vi "GenTargetGait.vi"() -> ()   [LabVIEW 2016]
uses:
  Sim&Process/DataProcess/CAlex2-Data/CAlex2_Data.lvclass
  D:/JinXin/LabVIEW.git/CAlex2-Controller-master/Sim&Process/DataProcess/ExpData/ExpData.lvclass
  Sim&Process/DataProcess/CAlex2-Data/PropertyNodes/Get_JointAngles.vi
  <vilib>/Utility/file.llb/Write Delimited Spreadsheet (string).vi
  <vilib>/Utility/file.llb/Write Delimited Spreadsheet (DBL).vi
  Sim&Process/DataProcess/ExpData/ExpData.lvclass
  <vilib>/GoldZinc Software/auzn custom VIs/CustomVI.lvlib
panel:
  out "AveragedJointAngle":dbl[][](array[numeric])
  out "TargetJointAngle":dbl[][](array[numeric])
  out "TargetTraj":dbl[][](array[numeric])
  in  "Save":bool
  in  "ScalingCoef Knee":dbl=1.0 format="%#_13g"
  out "Leg Length":cluster{"Thigh":dbl, "Shank":dbl}
  in  "Scale Method":enum16{"GaitHeight", "Angle"}(ring)
  in  "OutputLength":i32=500
  in  "ScalingCoef Hip":dbl=1.3 format="%#_13g"
  out "Array":dbl[](array[numeric])
  in  "Update":bool
  in  "Open":bool
  in  "stop":bool
  in  "EndTime":dbl=240.0
  in  "StartTime":dbl=60.0
  in  "Cut":bool
  out "AveragedTrajectory":dbl[][](graph)
  out "Averaged":cluster{"Mean":dbl[], "Mean":dbl[]}[](graph)
  out "Stacked":T1(graph)
  out "Ankle - X":dbl[][](graph)
  in  "Cut Parameter":dbl=100.0
  in  "Path":path
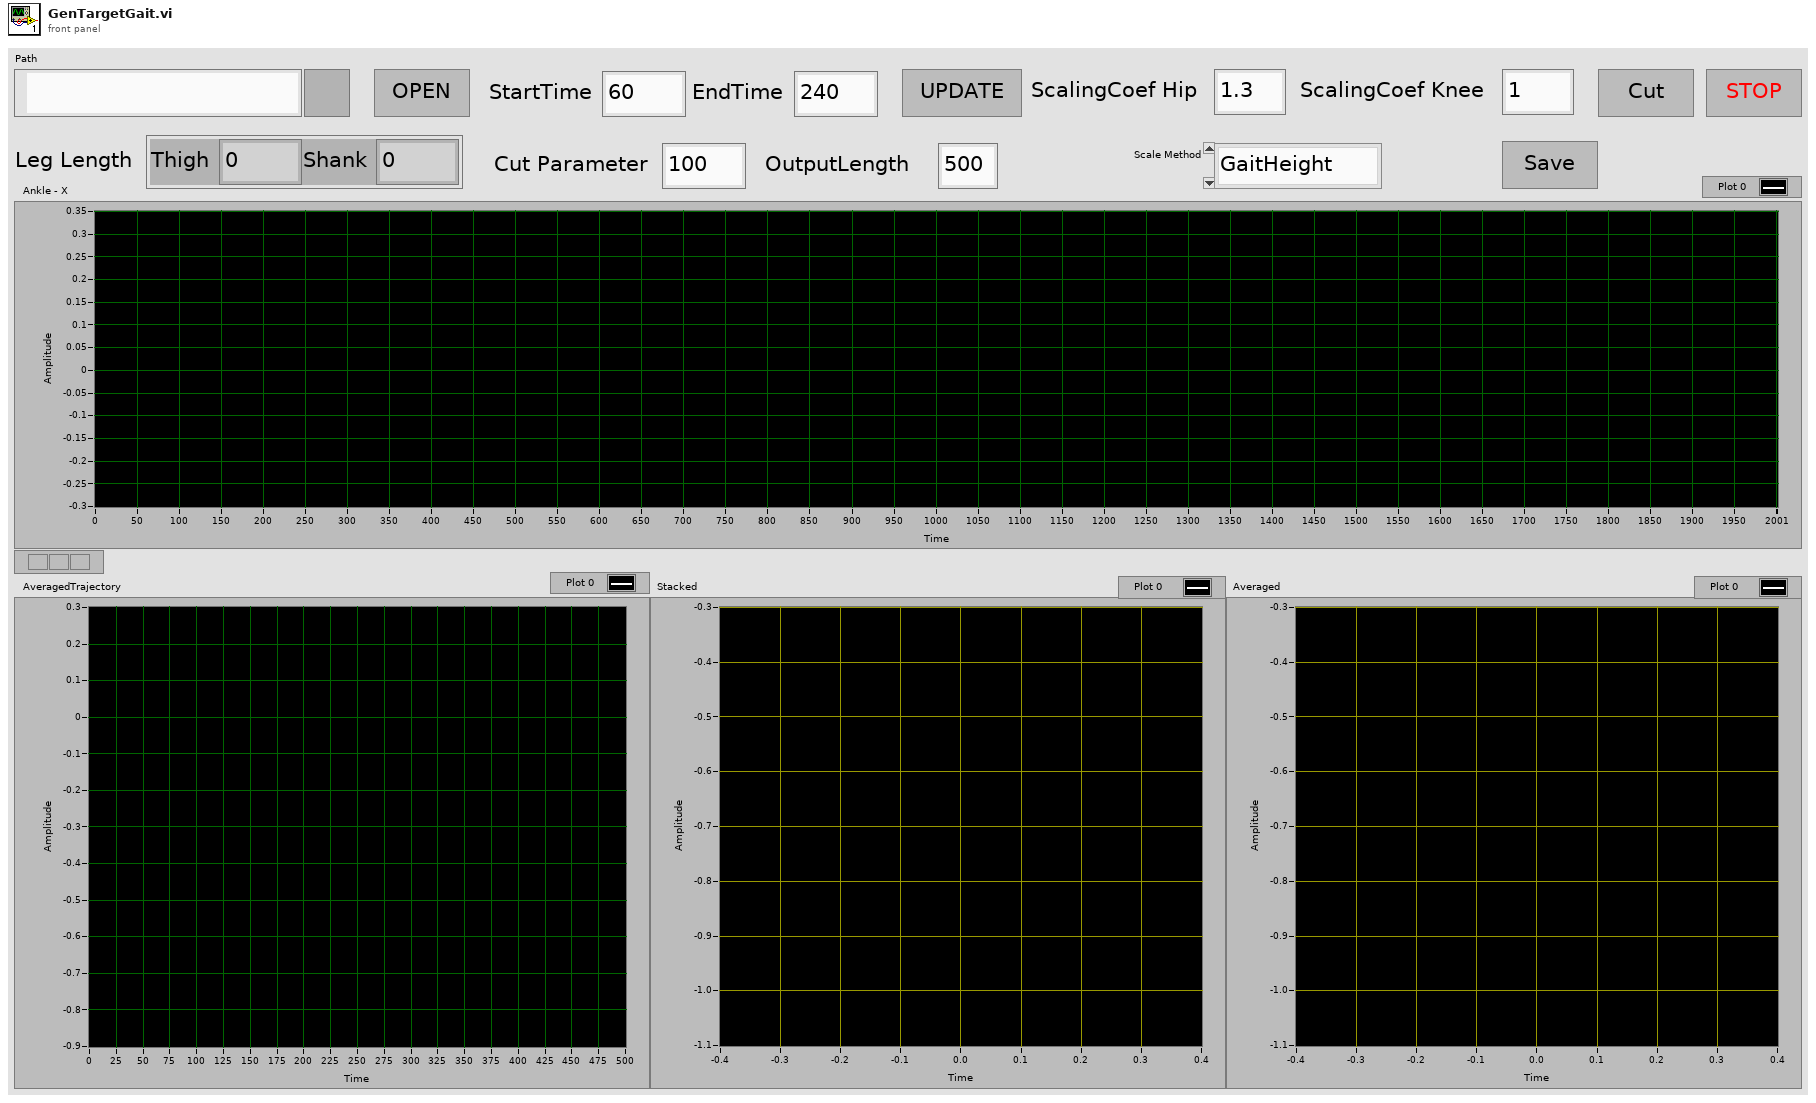
[diagram p1: front panel]
types:
  T1 = cluster{"DataAccess:WaistPosition":dbl[], "DataAccess:WaistPosition":dbl[]}
  T2 = enum16{"open", "replace", "create", "open or create", "replace or create", "replace or create with confirmation"}
  T3 = cluster{"ThighLt":dbl, "ShankLt":dbl, "HipWd":dbl}
  T4 = cluster{"ScaledGait":dbl[], "ScaledGait":dbl[]}[]
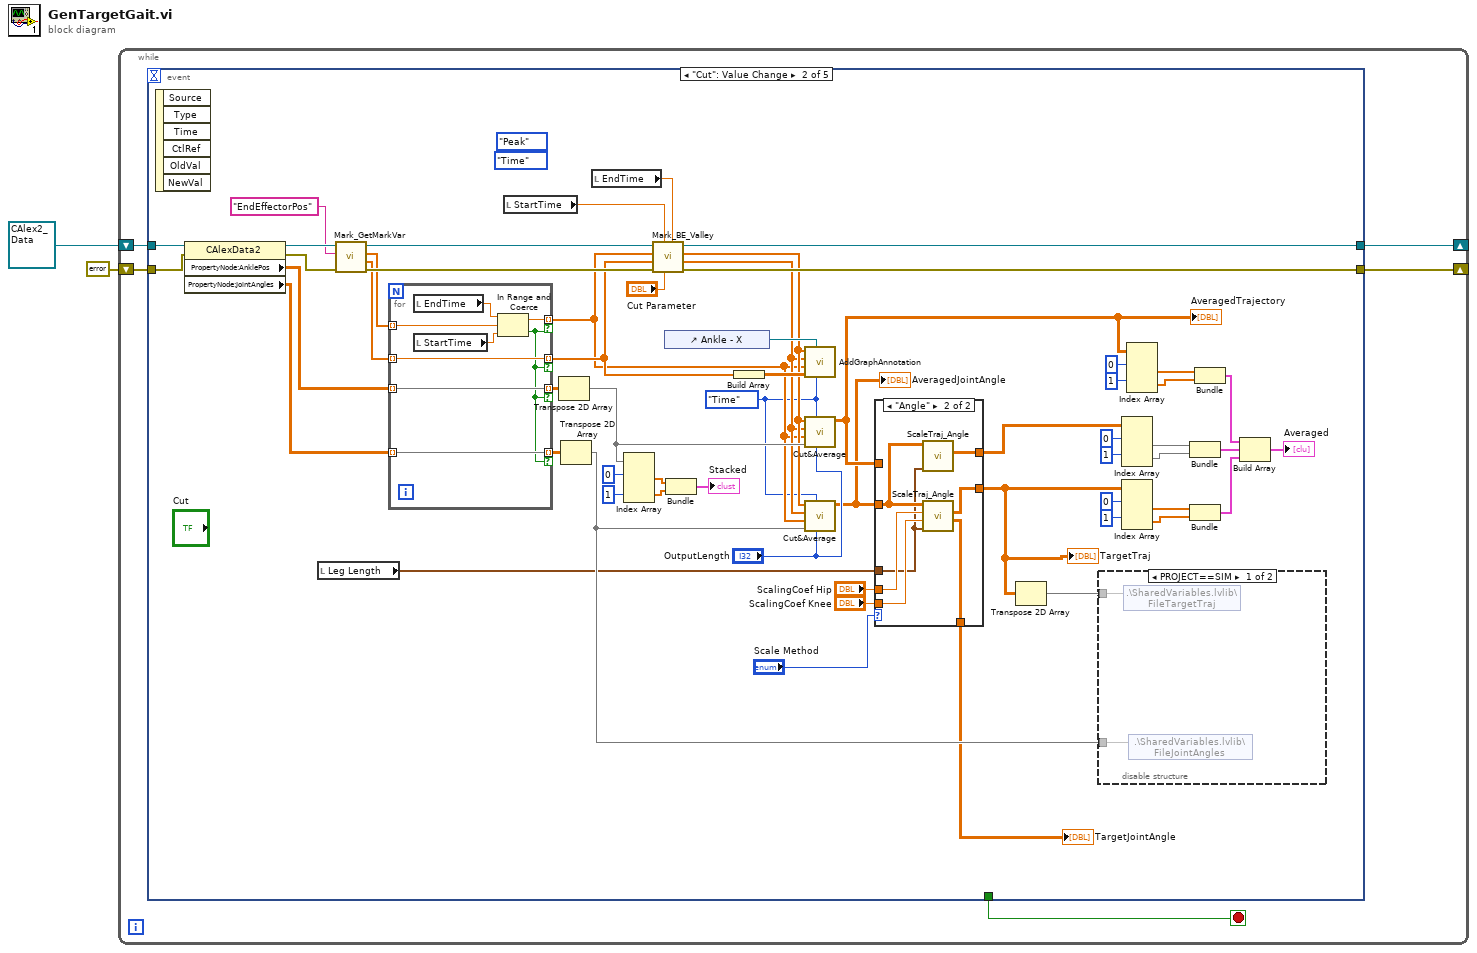
[diagram p0: block diagram]
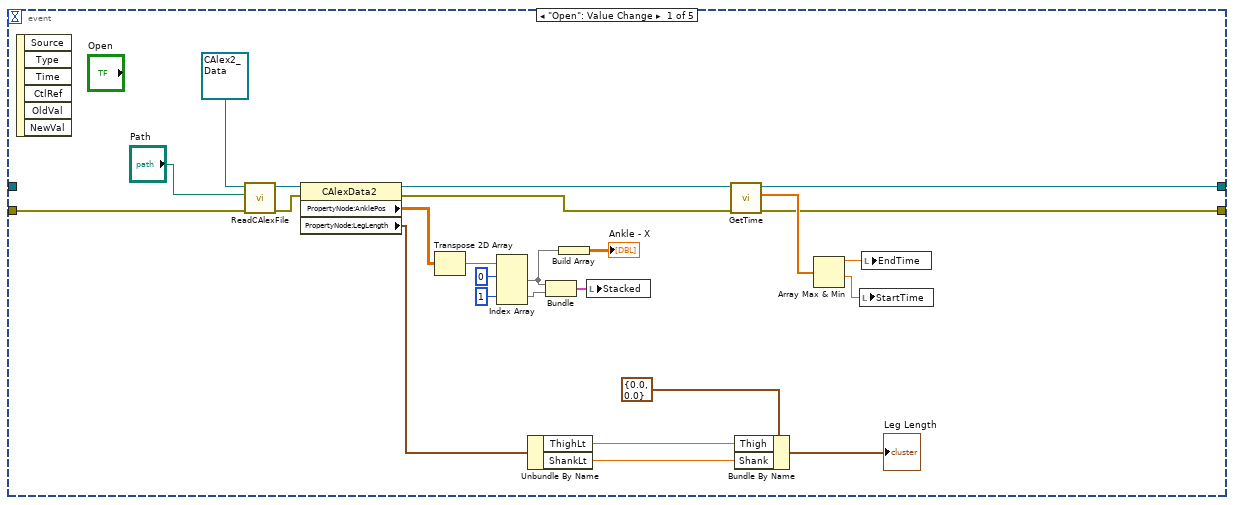
[diagram p2: hidden frame]
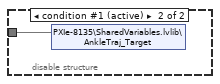
[diagram p3: hidden frame]
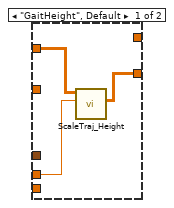
[diagram p4: hidden frame]
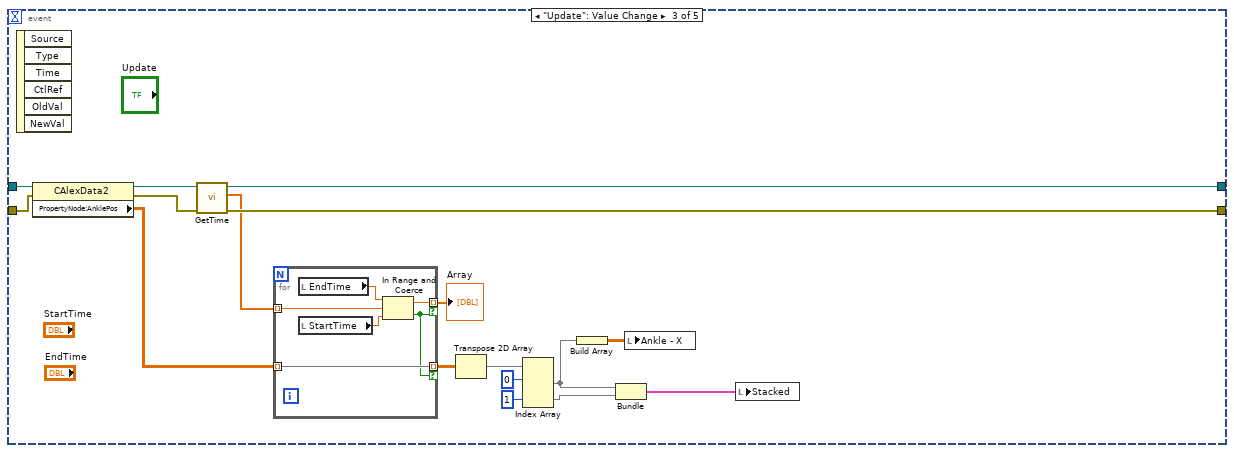
[diagram p5: hidden frame]
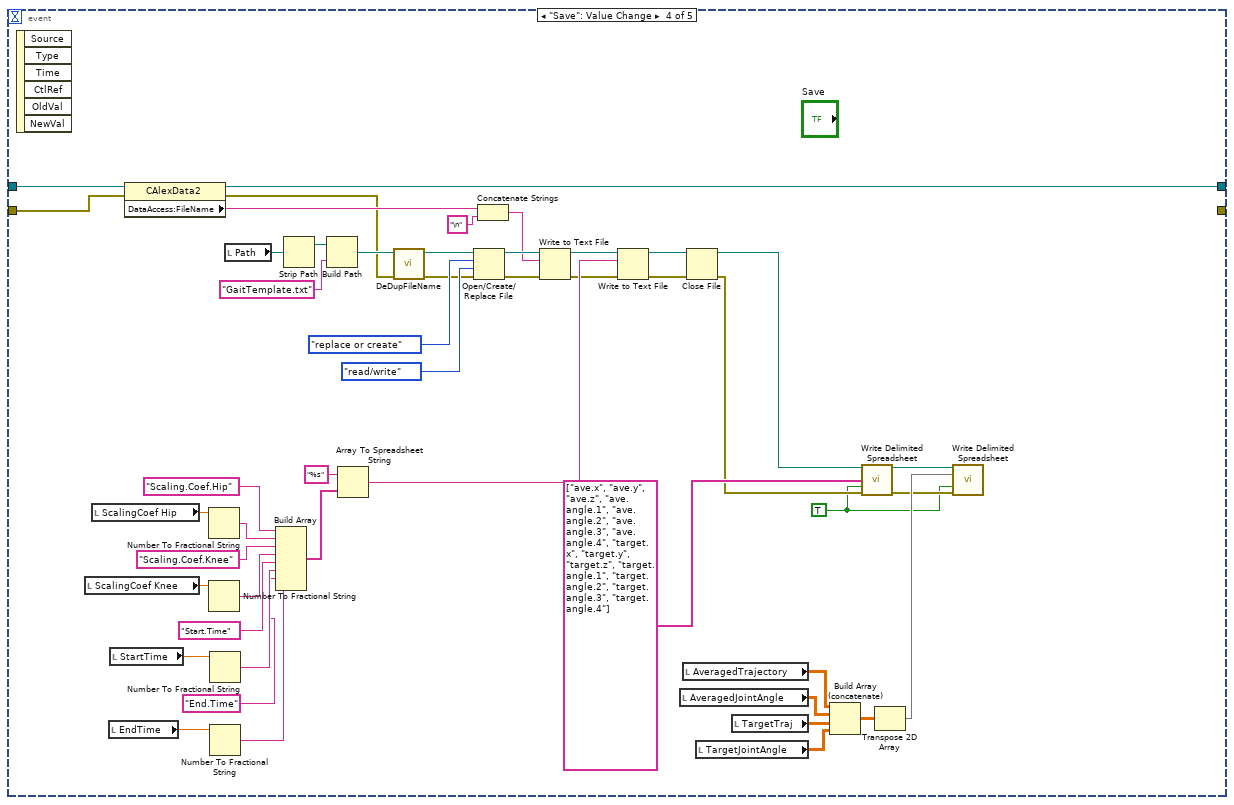
[diagram p6: hidden frame]
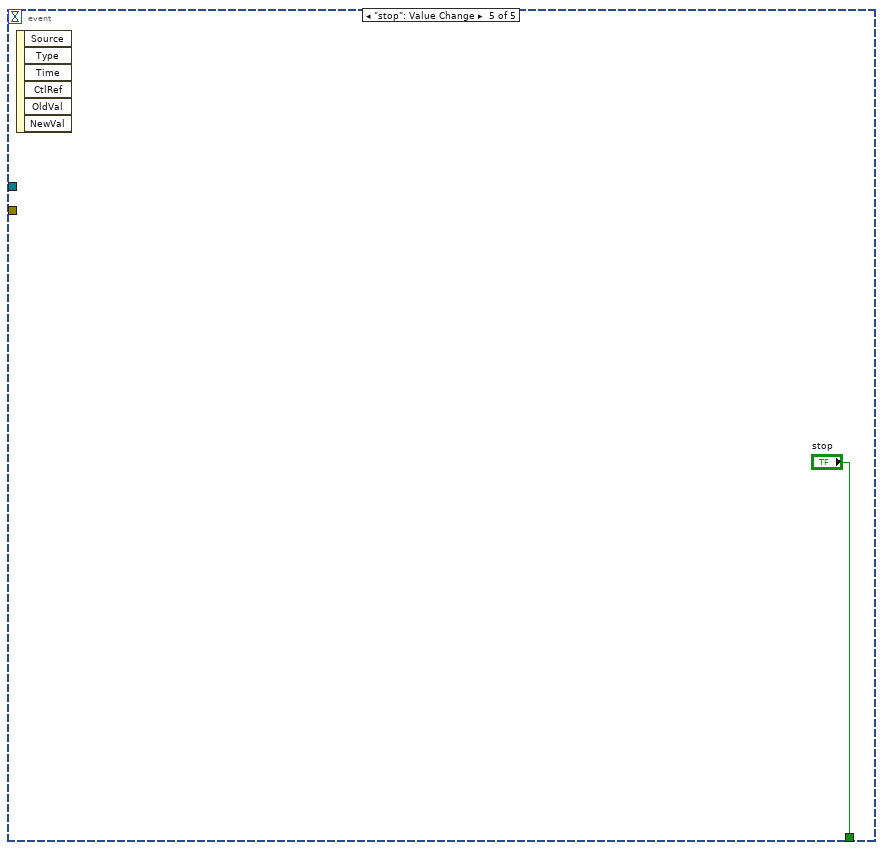
[diagram p7: hidden frame]
diagram:
  n1 = while {
    shift-right: [w4] -> _
    shift-left: refnum<class "CAlex2_Data.lvclass"> refnum ("CAlexData") -> [w7]
    shift-right: [w5] -> _
    shift-left: errorcluster {"status"=FALSE, "code"=0, "source"=""} ("error out") -> [w6]
    stop <- w3 stop-if-true
    n2 = event shown="[1] \"Cut\": Value Change" {
      selector: _ -> [_ _ _ _ _]
      dyn-events: _ -> [_ _ _ _ _]
      timeout: _ -> [_ _ _ _ _]
      tunnel: w7 -> [_ w83 w126 w148 _]
      tunnel: w6 -> [w22 w81 w125 w149 _]
      tunnel: [w19 w73 w117 _ _] -> w5
      tunnel: [w21 w72 w119 w147 _] -> w4
      tunnel: [_ _ _ _ "stop"] -> w3
      event "Open": Value Change {
        n3 = event-data() -> ()  [unwired: 1 in, 6 out]
        n4 = call "ReadCAlexFile.vi"("error in (no error)"=w22, "ExpData File Path"="Path", "CAlexData2"=refnum<class "CAlex2_Data.lvclass"> refnum ("CAlexData")) -> ("error out"=w16:errorcluster, "CAlexData 2"=w18:refnum<class "CAlex2_Data.lvclass">)  [unwired: 7 in]
        n5 = property class="CAlexData2"(reference=w18, error in=w16) -> (reference out=w17:refnum<class "CAlex2_Data.lvclass">, error out=w15:errorcluster, "PropertyNode:AnklePos"=w14:dbl[][], "PropertyNode:LegLength"=w13:T3)
        n6 = Transpose 2D Array(2D array=w14) -> (transposed array=w8:dbl[][])
        n7 = Index Array(array=w8, index (row) #1=0 ("index (row)"), index (row) #2=1 ("index (row)")) -> (element #1=w26:dbl[], element #2=w25:dbl[])  [unwired: 2 in]
        n8 = Unbundle By Name(w13) -> ("ThighLt"=w11:dbl, "ShankLt"=w10:dbl)
        n9 = Bundle(w26, w25) -> (w28:cluster{dbl[], dbl[]})  [unwired: 1 in]
        n10 = Build Array(w26) -> (→"Ankle - X":dbl[][])
        n11 = local write "Stacked"(w28) -> ()
        n12 = call "GetTime.vi"("error in (no error)"=w15, "CarexMData in"=w17) -> ("error out"=w19:errorcluster, "Time"=w20:dbl[], "CarexMData out"=w21:refnum<class "CAlex2_Data.lvclass">)  [unwired: 7 in]
        n13 = Bundle By Name(cluster=cluster{"Thigh":dbl, "Shank":dbl} {"Thigh"=0.0, "Shank"=0.0} ("Leg Length"), "Thigh"=w11, "Shank"=w10) -> (→"Leg Length":cluster{"Thigh":dbl, "Shank":dbl})
        n14 = Array Max & Min(array=w20) -> (max value=w32:dbl, min value=w31:dbl)  [unwired: 2 out]
        n15 = local write "StartTime"(w31) -> ()
        n16 = local write "EndTime"(w32) -> ()
      }
      event "Cut": Value Change {
        w66 = enum16{"Time", "Percentage", "Index"}."Time" ("Input Type")
        (unwired) enum16{"Peak", "Valley"}."Peak" ("Peak/Valley")
        (unwired) enum16{"Time", "Percentage", "Index"}."Time" ("Output Type")
        n17 = event-data() -> ()  [unwired: 1 in, 6 out]
        n18 = property class="CAlexData2"(reference=w83, error in=w81) -> (reference out=w82:refnum<class "CAlex2_Data.lvclass">, error out=w80:errorcluster, "PropertyNode:AnklePos"=w36:dbl[][], "PropertyNode:JointAngles"=w35:dbl[][])
        n19 = local read "Leg Length"() -> (w38:cluster{"Thigh":dbl, "Shank":dbl})
        n20 = call "Mark_GetMarkVar.vi"("error in (no error)"=w80, "VarName"="EndEffectorPos", "ExpData in"=w82) -> ("error out"=w90:errorcluster, "Var"=w88:dbl[], "Time"=w89:dbl[], "ExpData out"=w84:refnum<class "CAlex2_Data.lvclass">)  [unwired: 4 in, 1 out]
        n21 = for {
          tunnel: w89 -> [w112] mode=indexing
          tunnel: w88 -> [w108] mode=indexing
          tunnel: [w109] -> w68 mode=indexing if=w105
          tunnel: [w108] -> w87 mode=indexing if=w105
          tunnel: w36 -> [w107] mode=indexing
          tunnel: [w107] -> w79 mode=indexing if=w105
          tunnel: w35 -> [w106] mode=indexing
          tunnel: [w106] -> w61 mode=indexing if=w105
          n22 = local read "EndTime"() -> (w110:dbl)
          n23 = local read "StartTime"() -> (w111:dbl)
          n24 = In Range and Coerce(upper limit=w110, x=w112, lower limit=w111) -> (coerced(x)=w109:dbl, In Range?=w105:bool)
        }
        n25 = local read "StartTime"() -> (w33:dbl)
        n26 = Transpose 2D Array(2D array=w79) -> (transposed array=w71:dbl[][])
        n27 = Transpose 2D Array(2D array=w61) -> (transposed array=w48:dbl[][])
        n28 = local read "EndTime"() -> (w34:dbl)
        n29 = Index Array(array=w71, index (row) #1=0 ("index (row)"), index (row) #2=1 ("index (row)")) -> (element #1=w76:dbl[], element #2=w75:dbl[])  [unwired: 2 in]
        n30 = call "Mark_BE_Valley.vi"("End Time"=w34, "HalfWidth"="Cut Parameter", "Start Time"=w33, "error in (no error)"=w90, "Input"=w87, "Time"=w68, "CarexData In"=w84) -> ("error out"=w73:errorcluster, "End"=w69:dbl[], "Begin"=w70:dbl[], "CarexData Out"=w72:refnum<class "CAlex2_Data.lvclass">)  [unwired: 1 in]
        n31 = control-ref of="Ankle - X"() -> (w85:refnum<vi>)
        n32 = Bundle(w76, w75) -> (→"Stacked":cluster{dbl[], dbl[]})  [unwired: 1 in]
        n33 = Build Array(w87) -> (w86:dbl[][])
        n34 = call <vilib>:"AddGraphAnnotation.vi"("Input Type (Time)"=w66, "WaveformGraph in"=w85, "Array"=w86, "Time"=w68, "Valleys  (Yellow)"=w69, "Peaks (Red)"=w70) -> ()  [unwired: 4 in, 2 out]
        n35 = call <vilib>:"Cut&Average.vi"("Dilate Length (200)"="OutputLength", "Input Type (Time)"=w66, "Data"=w71, "Time"=w68, "End"=w69, "Begin"=w70) -> ("Mean"=w52:dbl[][])  [unwired: 5 out]
        "AveragedTrajectory" <- w52
        n36 = call <vilib>:"Cut&Average.vi"("Dilate Length (200)"="OutputLength", "Input Type (Time)"=w66, "Data"=w48, "Time"=w68, "End"=w69, "Begin"=w70) -> ("Mean"=w47:dbl[][])  [unwired: 5 out]
        "AveragedJointAngle" <- w47
        n37 = case shown="\"Angle\"" "Scale Method" {
          tunnel: [w96 w103] -> w49
          tunnel: w47 -> [_ w100]
          tunnel: w38 -> [_ w99]
          tunnel: "ScalingCoef Hip" -> [w97 w104]
          tunnel: w52 -> [w95 _]
          tunnel: "ScalingCoef Knee" -> [_ w102]
          tunnel: [_ w101] -> w46
          tunnel: [_ w98] -> w41
          frame "GaitHeight", Default {
            n38 = call "ScaleTraj_Height.vi"("ScalingCoef"=w97, "Averaged Gait"=w95) -> ("ScaledGait"=w96:dbl[][])  [unwired: 8 in, 1 out]
          }
          frame "Angle" {
            n39 = call "ScaleTraj_Angle.vi"("ArmLength"=w99, "AverageJointAngles"=w100) -> ("ScaledGait"=w98:dbl[][])  [unwired: 8 in, 1 out]
            n40 = call "ScaleTraj_Angle.vi"("ArmLength"=w99, "ScalingCoef Knee (1)"=w102, "ScalingCoef Hip (1)"=w104, "AverageJointAngles"=w100) -> ("ScaledJointAngles"=w101:dbl[][], "ScaledGait"=w103:dbl[][])  [unwired: 6 in]
          }
        }
        "TargetTraj" <- w49
        "TargetJointAngle" <- w46
        n41 = Transpose 2D Array(2D array=w49) -> (transposed array=w51:dbl[][])
        n42 = disable-structure shown="PROJECT==SIM" {
          disable-tunnel: w51 -> [w93 w94]
          disable-tunnel: w48 -> [w92 _]
          frame condition #0 {
            n43 = shared-variable ".\\SharedVariables.lvlib\\FileTargetTraj"(w93) -> ()  [unwired: 1 in, 1 out]
            n44 = shared-variable ".\\SharedVariables.lvlib\\FileJointAngles"(w92) -> ()  [unwired: 1 in, 1 out]
          }
          frame condition #1 (active) {
            n45 = shared-variable "PXIe-8135\\SharedVariables.lvlib\\AnkleTraj_Target"(w94) -> ()  [unwired: 1 in, 1 out]
          }
        }
        n46 = Index Array(array=w41, index (row) #1=0 ("index (row)"), index (row) #2=1 ("index (row)")) -> (element #1=w43:dbl[], element #2=w42:dbl[])  [unwired: 2 in]
        n47 = Index Array(array=w49, index (row) #1=0 ("index (row)"), index (row) #2=1 ("index (row)")) -> (element #1=w63:dbl[], element #2=w62:dbl[])  [unwired: 2 in]
        n48 = Index Array(array=w52, index (row) #1=0 ("index (row)"), index (row) #2=1 ("index (row)")) -> (element #1=w57:dbl[], element #2=w58:dbl[])  [unwired: 2 in]
        n49 = Bundle("ScaledGait"=w43, "ScaledGait"=w42) -> (w39:cluster{"ScaledGait":dbl[], "ScaledGait":dbl[]})  [unwired: 1 in]
        n50 = Bundle("ScaledGait"=w63, "ScaledGait"=w62) -> (w54:cluster{"ScaledGait":dbl[], "ScaledGait":dbl[]})  [unwired: 1 in]
        n51 = Bundle("Mean"=w57, "Mean"=w58) -> (w40:cluster{"Mean":dbl[], "Mean":dbl[]})  [unwired: 1 in]
        n52 = Build Array(w40, w39, w54) -> (→"Averaged":T4)
      }
      event "Update": Value Change {
        n53 = event-data() -> ()  [unwired: 1 in, 6 out]
        n54 = property class="CAlexData2"(reference=w126, error in=w125) -> (reference out=w120:refnum<class "CAlex2_Data.lvclass">, error out=w118:errorcluster, "PropertyNode:AnklePos"=w115:dbl[][])
        n55 = call "GetTime.vi"("error in (no error)"=w118, "CarexMData in"=w120) -> ("error out"=w117:errorcluster, "Time"=w116:dbl[], "CarexMData out"=w119:refnum<class "CAlex2_Data.lvclass">)  [unwired: 7 in]
        n56 = for {
          tunnel: w116 -> [w135] mode=indexing
          tunnel: [w132] -> w124 mode=indexing if=w130
          tunnel: w115 -> [w131] mode=indexing
          tunnel: [w131] -> w114 mode=indexing if=w130
          n57 = local read "EndTime"() -> (w133:dbl)
          n58 = local read "StartTime"() -> (w134:dbl)
          n59 = In Range and Coerce(upper limit=w133, x=w135, lower limit=w134) -> (coerced(x)=w132:dbl, In Range?=w130:bool)
        }
        "Array" <- w124
        n60 = Transpose 2D Array(2D array=w114) -> (transposed array=w113:dbl[][])
        n61 = Index Array(array=w113, index (row) #1=0 ("index (row)"), index (row) #2=1 ("index (row)")) -> (element #1=w122:dbl[], element #2=w121:dbl[])  [unwired: 2 in]
        n62 = Build Array(w122) -> (w123:dbl[][])
        n63 = Bundle(w122, w121) -> (w127:cluster{dbl[], dbl[]})  [unwired: 1 in]
        n64 = local write "Ankle - X"(w123) -> ()
        n65 = local write "Stacked"(w127) -> ()
      }
      event "Save": Value Change {
        w136 = TRUE ("append to file? (new file:F)")
        n66 = event-data() -> ()  [unwired: 1 in, 6 out]
        n67 = local read "ScalingCoef Knee"() -> (w174:dbl)
        n68 = local read "ScalingCoef Hip"() -> (w175:dbl)
        n69 = local read "EndTime"() -> (w159:dbl)
        n70 = local read "StartTime"() -> (w158:dbl)
        n71 = property class="CAlexData2"(reference=w148, error in=w149) -> (reference out=w147:refnum<class "CAlex2_Data.lvclass">, error out=w137:errorcluster, "DataAccess:FileName"=w146:string)
        n72 = Number To Fractional String(number=w175) -> (F-format string=w172:string)  [unwired: 3 in]
        n73 = Number To Fractional String(number=w174) -> (F-format string=w170:string)  [unwired: 3 in]
        n74 = Number To Fractional String(number=w158) -> (F-format string=w156:string)  [unwired: 3 in]
        n75 = Number To Fractional String(number=w159) -> (F-format string=w154:string)  [unwired: 3 in]
        n76 = local read "Path"() -> (w183:path)
        n77 = Build Array("Scaling.Coef.Hip" ("name or relative path"), w172, "Scaling.Coef.Knee" ("name or relative path"), w170, "Start.Time" ("name or relative path"), w156, "End.Time" ("name or relative path"), w154) -> (w169:string[])
        n78 = Strip Path(path=w183) -> (stripped path=w181:path)  [unwired: 1 out]
        n79 = Build Path(base path=w181, name or relative path="GaitTemplate.txt") -> (appended path=w140:path)
        n80 = Array To Spreadsheet String(array=w169, 3:"%s" ("format string")) -> (spreadsheet string=w168:string)  [unwired: 1 in]
        n81 = call <vilib>:"DeDupFileName.vi"("error in (no error)"=w137, "Path"=w140) -> ("error out"=w138:errorcluster, "Out Path"=w139:path)  [unwired: 7 in, 1 out]
        n82 = Open/Create/Replace File(file path (use dialog)=w139, error in=w138, operation (0:open)=T2."replace or create", access (0:read/write)=enum16{"read/write", "read-only", "write-only"}."read/write") -> (refnum out=w153:refnum<file>, error out=w151:errorcluster)  [unwired: 2 in, 1 out]
        n83 = Concatenate Strings(w146, "\n" ("string")) -> (w145:string)
        n84 = Write to Text File(file (use dialog)=w153, text=w145, error in=w151) -> (refnum out=w152:refnum<file>, error out=w150:errorcluster)  [unwired: 1 in, 1 out]
        n85 = Write to Text File(file (use dialog)=w152, text=w168, error in=w150) -> (refnum out=w164:refnum<file>, error out=w165:errorcluster)  [unwired: 1 in, 1 out]
        n86 = local read "AveragedJointAngle"() -> (w161:dbl[][])
        n87 = local read "AveragedTrajectory"() -> (w162:dbl[][])
        n88 = Close File(refnum=w164, error in=w165) -> (path=w163:path, error out=w142:errorcluster)
        n89 = local read "TargetJointAngle"() -> (w179:dbl[][])
        n90 = local read "TargetTraj"() -> (w182:dbl[][])
        n91 = Build Array (concatenate)(w162, w161, w182, w179) -> (w178:dbl[][])
        n92 = call-poly <vilib>:"Write Delimited Spreadsheet.vi"("file path (dialog if empty)"=w163, "1D data"=string[] ["ave.x", "ave.y", "ave.z", "ave.angle.1", "ave.angle.2", "ave.angle.3", "ave.angle.4", "target.x", "target.y", "target.z", "target.angle.1", "target.angle.2", "target.angle.3", "target.angle.4"], "append to file? (new file:F)"=w136, "error in (no error)"=w142) -> ("new file path (Not A Path if cancelled)"=w177:path, "error out"=w141:errorcluster)  [unwired: 10 in]
        n93 = Transpose 2D Array(2D array=w178) -> (transposed array=w176:dbl[][])
        n94 = call-poly <vilib>:"Write Delimited Spreadsheet.vi"("file path (dialog if empty)"=w177, "2D data"=w176, "append to file? (new file:F)"=w136, "error in (no error)"=w141) -> ()  [unwired: 10 in, 2 out]
      }
      event "stop": Value Change {
        n95 = event-data() -> ()  [unwired: 1 in, 6 out]
      }
    }
  }
